vi "PH_Sequencer.set Voltage Knobs visible.vi"(0 "VI in":refnum<vi>, 5 "error in (no error)":errorcluster) -> (14 "VI out":refnum<vi>, 19 "error out":errorcluster)   [LabVIEW 2014, in "PH_Sequencer.lvlib"]
doc: "This VI sets the voltage selectors to be en- or disabled."
uses:
  PH_Sequencer.lvlib
  PH_Basics/PH_PP_Common/PH_PP_Common.PUs.ctl
  PH_BeamlineInformation/PH_BeamlineInformation.lvlib
  PH_Basics/PH_PP_Common/PH_PP_Common.lvlib
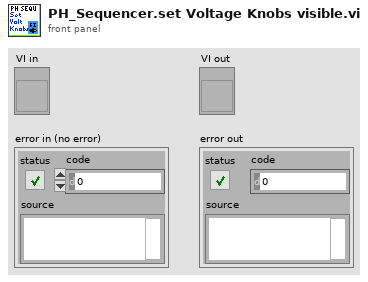
[diagram p1: front panel]
types:
  T1 = typedef "PH_PP_Common.lvlib/PH_PP_Common.PUs.ctl" = enum16{"no Info", "PA-19mm-1", "PA-19mm-2", "PA-45mm-PILC", "PA-45mm-MAIN", "MA-PU-1", "MA-PU-2", "MA-PU-3", "MA-PU-4", "MA-PU-5", "MA-PU-6", "MA-FR", "MA-PILC", "PA-45mm-DP"}
  T2 = typedef "PH_BeamlineInformation.lvlib/PH_BeamlineInformation.i attribute.ctl" = cluster{"BL GUI Elements of Services":cluster{"Service Name":string, "GUI Elements":refnum<vi>[], "Status":i32}[], "Powermeters":T3, "Efficiency":T4, "Heads":T5[]}
  T3 = typedef "PH_BeamlineInformation.lvlib/PH_BeamlineInformation.Powermeter.ctl" = cluster{"ns FE":cluster{"GUI Ref":refnum<vi>, "Value":dbl}, "fs FE":cluster{"GUI Ref":refnum<vi>, "Value":dbl}, "PA":cluster{"GUI Ref":refnum<vi>, "Value":dbl}, "MA":cluster{"GUI Ref":refnum<vi>, "Value":dbl}, "Z6 green":cluster{"GUI Ref":refnum<vi>, "Value":dbl}, "Z6 IR":cluster{"GUI Ref":refnum<vi>, "Value":dbl}, "Z6 COS":cluster{"GUI Ref":refnum<vi>, "Value":dbl}}
  T4 = typedef "PH_BeamlineInformation.lvlib/PH_BeamlineInformation.Efficiency.ctl" = cluster{"PA Gain":cluster{"GUI Ref":refnum<vi>, "Value":dbl}, "MA Gain":cluster{"GUI Ref":refnum<vi>, "Value":dbl}, "Z6 green Conversion":cluster{"GUI Ref":refnum<vi>, "Value":dbl}, "Z6 Comp Losses":cluster{"GUI Ref":refnum<vi>, "Value":dbl}}
  T5 = typedef "PH_BeamlineInformation.lvlib/PH_BeamlineInformation.Head.ctl" = cluster{"PowerUnit":T1, "in use":cluster{"Value":bool, "GUI Ref":refnum<vi>, "linked":bool}, "voltage":cluster{"Value":dbl, "GUI Ref":refnum<vi>, "linked":bool}}
  T6 = enum8{"Enabled", "Disabled", "Disabled and Grayed Out"}
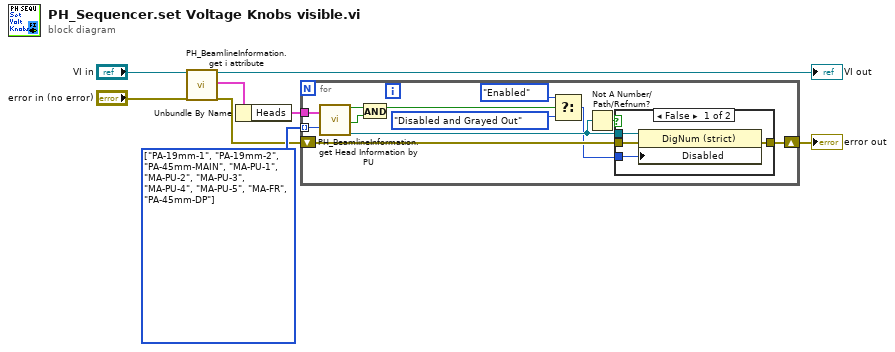
[diagram p0: block diagram]
diagram:
  w8 = T1[] [enum."PA-19mm-1", enum."PA-19mm-2", enum."PA-45mm-MAIN", enum."MA-PU-1", enum."MA-PU-2", enum."MA-PU-3", enum."MA-PU-4", enum."MA-PU-5", enum."MA-FR", enum."PA-45mm-DP"] items=["no Info", "PA-19mm-1", "PA-19mm-2", "PA-45mm-PILC", "PA-45mm-MAIN", "MA-PU-1", "MA-PU-2", "MA-PU-3", "MA-PU-4", "MA-PU-5", "MA-PU-6", "MA-FR", "MA-PILC", "PA-45mm-DP"]
  n1 = call "PH_BeamlineInformation.get i attribute.vi"("i ref in"="VI in", "error in (no error)"="error in (no error)") -> ("i ref out"=→"VI out":refnum<vi>, "i attribute"=w4:T2, "error out"=w3:errorcluster)  [unwired: 15 in]
  n2 = Unbundle By Name(w4) -> ("Heads"=w7:T5[])
  n3 = for {
    shift-right: [w18] -> w6
    shift-left: w3 -> [w19]
    tunnel: w7 -> [w16]
    tunnel: w8 -> [w15] mode=indexing
    n4 = call "PH_BeamlineInformation.get Head Information by PU.vi"("Heads"=w16, "Power Unit"=w15) -> ("In Use?"=w14:bool, "Voltage linked?"=w9:bool, "Voltage GUI Ref"=w17:refnum<vi>)  [unwired: 12 in, 3 out]
    n5 = And(x=w14, y=w9) -> (x .and. y?=w10:bool)
    n6 = Select(t=T6."Enabled" ("Disabled"), s=w10, f=T6."Disabled and Grayed Out") -> (s? t:f=w13:T6)
    n7 = Not A Number/Path/Refnum?(number/path/refnum=w17) -> (NaN/Path/Refnum?=w20:bool)
    n8 = case shown="False" w20 {
      tunnel: w17 -> [w24 _]
      tunnel: w19 -> [w23 w25]
      tunnel: [w22 w25] -> w18
      tunnel: w13 -> [w21 _]
      frame False {
        n9 = property class="DigNum (strict)"(reference=w24, error in=w23, "Disabled"=w21) -> (error out=w22:errorcluster)  [unwired: 1 out]
      }
      frame True {
      }
    }
  }
  "error out" <- w6
